vi "Send Status Complete.vi"(8 "Error In":errorcluster, 9 "Grader Result":T6, 10 "Challenge Config":T5, 11 "VIChallenge Config in":T1) -> (0 "Error Out":errorcluster, 3 "VIChallenge Config":T1)   [LabVIEW 2013, in "VIChallenge.lvlib"]
doc: "Send job complete status along with pass / fail status, score, and scoresort order."
uses:
  <vilib>/LabVIEW Hacker/VIChallenge/VIChallenge.lvlib
  <vilib>/LabVIEW Hacker/VIChallenge/Private/Grader/Type Defs/Grader Result.ctl
  <vilib>/LabVIEW Hacker/VIChallenge/Private/Type Defs/Database/Score.ctl
  <vilib>/LabVIEW Hacker/VIChallenge/Private/Grader/Type Defs/UTF Status.ctl
  <vilib>/LabVIEW Hacker/VIChallenge/Private/Grader/Type Defs/Challenge.ctl
  <vilib>/LabVIEW Hacker/VIChallenge/Private/Type Defs/VIChallenge Config.ctl
  <vilib>/National Instruments/NI Amazon Web Services (AWS) Toolkit for LabVIEW/SQS/VI Source/AWS SQS Class/AWS_SQS.lvclass
  <vilib>/National Instruments/NI Amazon Web Services (AWS) Toolkit for LabVIEW/AWS Core Lib/VI Source/Typedefs/AWS_AWS Credentials.ctl
  <vilib>/LabVIEW Hacker/VIChallenge/Private/Type Defs/JSON_job.ctl
  <vilib>/addons/database/Connection.llb/Conn ObjectReference.ctl
  <vilib>/LabVIEW Hacker/VIChallenge/Private/Type Defs/JSON_job_complete_status.ctl
  <vilib>/National Instruments/NI Amazon Web Services (AWS) Toolkit for LabVIEW/SQS/VI Source/Public Typedefs/AWS_SQS SendMessage.ctl
  <vilib>/National Instruments/NI Amazon Web Services (AWS) Toolkit for LabVIEW/SQS/VI Source/AWS_SQS.lvlib
  <vilib>/National Instruments/NI Amazon Web Services (AWS) Toolkit for LabVIEW/AWS Core Lib/VI Source/AWS_Core.lvlib
  <vilib>/addons/database/NI_Database_API.lvlib
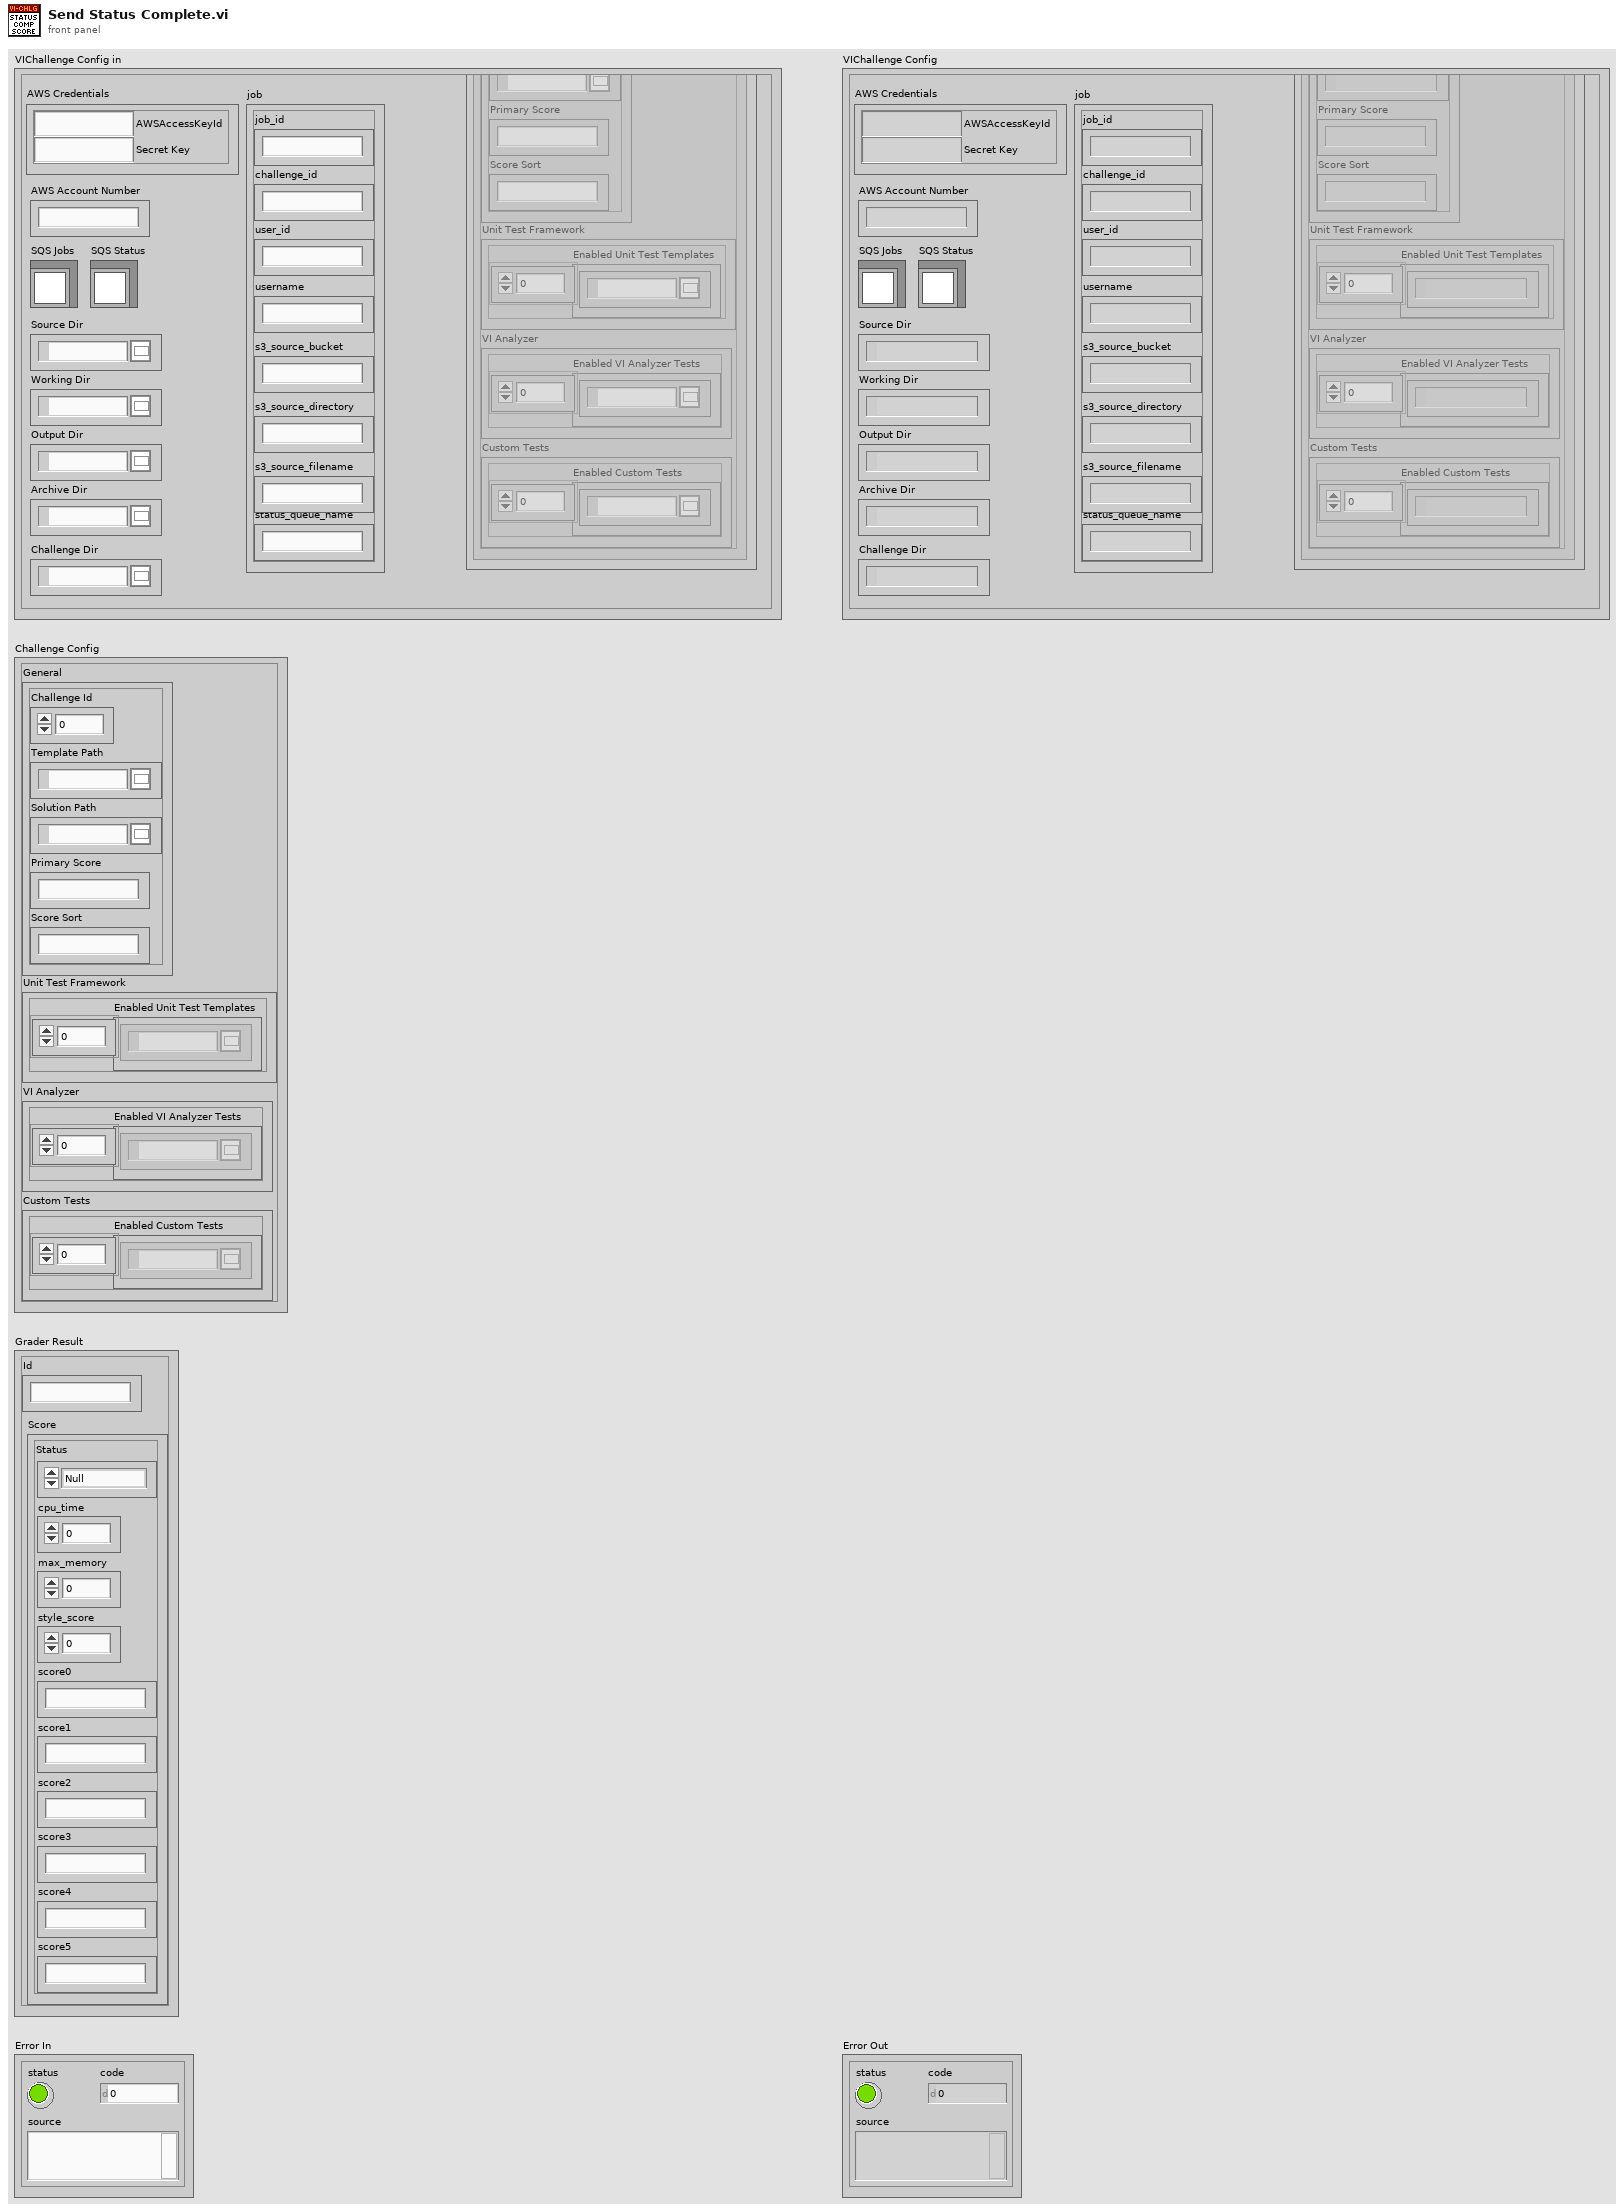
[diagram p1: front panel]
types:
  T1 = typedef "VIChallenge.lvlib/VIChallenge Config.ctl" = cluster{"AWS Credentials":T2, "AWS Account Number":string, "SQS Jobs":refnum<class "AWS_SQS.lvclass">, "SQS Status":refnum<class "AWS_SQS.lvclass">, "Source Dir":path, "Working Dir":path, "Output Dir":path, "Archive Dir":path, "job":T3, "Database Ref":T4, "Challenge Dir":path, "Challenges":T5[]}
  T2 = typedef "AWS_Core.lvlib/AWS_AWS Credentials.ctl" = cluster{"AWSAccessKeyId":string, "Secret Key":string}
  T3 = typedef "VIChallenge.lvlib/JSON_job.ctl" = cluster{"job_id":string, "challenge_id":string, "user_id":string, "s3_source_bucket":string, "s3_source_directory":string, "s3_source_filename":string, "status_queue_name":string, "username":string}
  T4 = typedef "NI_Database_API.lvlib/Conn ObjectReference.ctl" = refnum<k1>
  T5 = typedef "VIChallenge.lvlib/Challenge.ctl" = cluster{"General":cluster{"Challenge Id":i32, "Template Path":path, "Solution Path":path, "Primary Score":string, "Score Sort":string}, "Unit Test Framework":cluster{"Enabled Unit Test Templates":path[]}, "VI Analyzer":cluster{"Enabled VI Analyzer Tests":path[]}, "Custom Tests":cluster{"Enabled Custom Tests":path[]}}
  T6 = typedef "VIChallenge.lvlib/Grader Result.ctl" = cluster{"Id":string, "Score":T7}
  T7 = typedef "VIChallenge.lvlib/Score.ctl" = cluster{"Status":T8, "cpu_time":i32, "max_memory":i32, "style_score":i32, "score0":string, "score1":string, "score2":string, "score3":string, "score4":string, "score5":string}
  T8 = typedef "VIChallenge.lvlib/UTF Status.ctl" = enum16{"Null", "Passed", "Failed", "Error", "Skipped", "Not Processed"}
  T9 = typedef "AWS_SQS.lvlib/AWS_SQS SendMessage.ctl" = cluster{"MessageBody":string, "DelaySeconds":i32}
  T10 = typedef "VIChallenge.lvlib/JSON_job_complete_status.ctl" = cluster{"status":string, "details":cluster{"status":string, "score":string, "score_sort":string}}
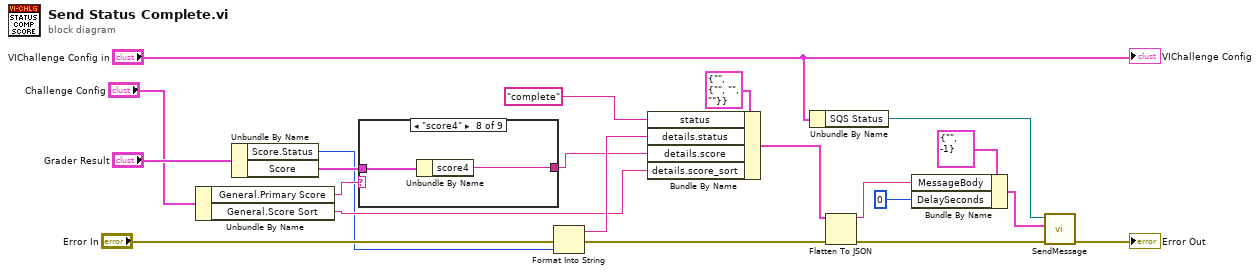
[diagram p0: block diagram]
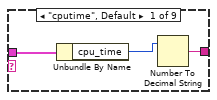
[diagram p2: hidden frame]
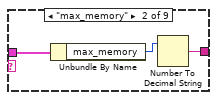
[diagram p3: hidden frame]
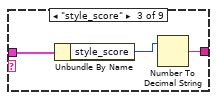
[diagram p4: hidden frame]
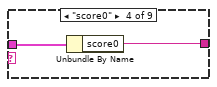
[diagram p5: hidden frame]
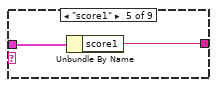
[diagram p6: hidden frame]
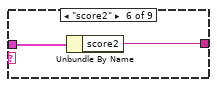
[diagram p7: hidden frame]
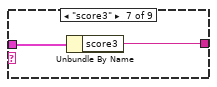
[diagram p8: hidden frame]
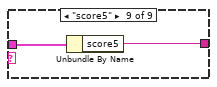
[diagram p9: hidden frame]
diagram:
  n1 = Unbundle By Name("Challenge Config") -> ("General.Primary Score"=w14:string, "General.Score Sort"=w13:string)
  n2 = Unbundle By Name("Grader Result") -> ("Score.Status"=w10:T8, "Score"=w20:T7)
  n3 = case shown="\"score4\"" w14 {
    tunnel: w20 -> [w24 w27 w30 w32 w34 w36 w38 w40 w42]
    tunnel: [w22 w25 w28 w31 w33 w35 w37 w39 w41] -> w16
    frame "cputime", Default {
      n4 = Unbundle By Name(w24) -> ("cpu_time"=w23:i32)
      n5 = Number To Decimal String(number=w23) -> (decimal integer string=w22:string)  [unwired: 1 in]
    }
    frame "max_memory" {
      n6 = Unbundle By Name(w27) -> ("max_memory"=w26:i32)
      n7 = Number To Decimal String(number=w26) -> (decimal integer string=w25:string)  [unwired: 1 in]
    }
    frame "style_score" {
      n8 = Unbundle By Name(w30) -> ("style_score"=w29:i32)
      n9 = Number To Decimal String(number=w29) -> (decimal integer string=w28:string)  [unwired: 1 in]
    }
    frame "score0" {
      n10 = Unbundle By Name(w32) -> ("score0"=w31:string)
    }
    frame "score1" {
      n11 = Unbundle By Name(w34) -> ("score1"=w33:string)
    }
    frame "score2" {
      n12 = Unbundle By Name(w36) -> ("score2"=w35:string)
    }
    frame "score3" {
      n13 = Unbundle By Name(w38) -> ("score3"=w37:string)
    }
    frame "score4" {
      n14 = Unbundle By Name(w40) -> ("score4"=w39:string)
    }
    frame "score5" {
      n15 = Unbundle By Name(w42) -> ("score5"=w41:string)
    }
  }
  n16 = Format Into String(error in="Error In", w10) -> (resulting string=w21:string, error out=w19:errorcluster)  [unwired: 2 in]
  n17 = Bundle By Name(cluster=T10 {"status"="", "details"={"status"="", "score"="", "score_sort"=""}} ("job_complete"), "status"="complete", "details.status"=w21, "details.score"=w16, "details.score_sort"=w13) -> (w17:T10)
  n18 = Unbundle By Name("VIChallenge Config in") -> ("SQS Status"=w9:refnum<class "AWS_SQS.lvclass">)
  n19 = Flatten To JSON(anything=w17, error in (no error)=w19) -> (JSON string=w4:string, 11:w2:errorcluster)  [unwired: 1 in]
  n20 = Bundle By Name(cluster=T9 {"MessageBody"="", "DelaySeconds"=-1} ("SendMessage Parameters"), "MessageBody"=w4, "DelaySeconds"=0) -> (w8:T9)
  n21 = call <vilib>:"SendMessage.vi"("error in (no error)"=w2, "SendMessage Parameters"=w8, "AWS_SQS.lvlib:AWS_SQS.lvclass"=w9) -> ("error out"=→"Error Out":errorcluster)  [unwired: 6 in, 2 out]
  "VIChallenge Config" <- "VIChallenge Config in"
